vi "videotest.vi"() -> ()   [LabVIEW 2014]
uses:
  <vilib>/userdefined/High Color/IMAQdx.ctl
  <vilib>/vision/driver/NI_Vision_Acquisition_Software.lvlib
panel:
  out "error out":errorcluster
  out "Image":T1(plugin-control)
  in  "stop":bool
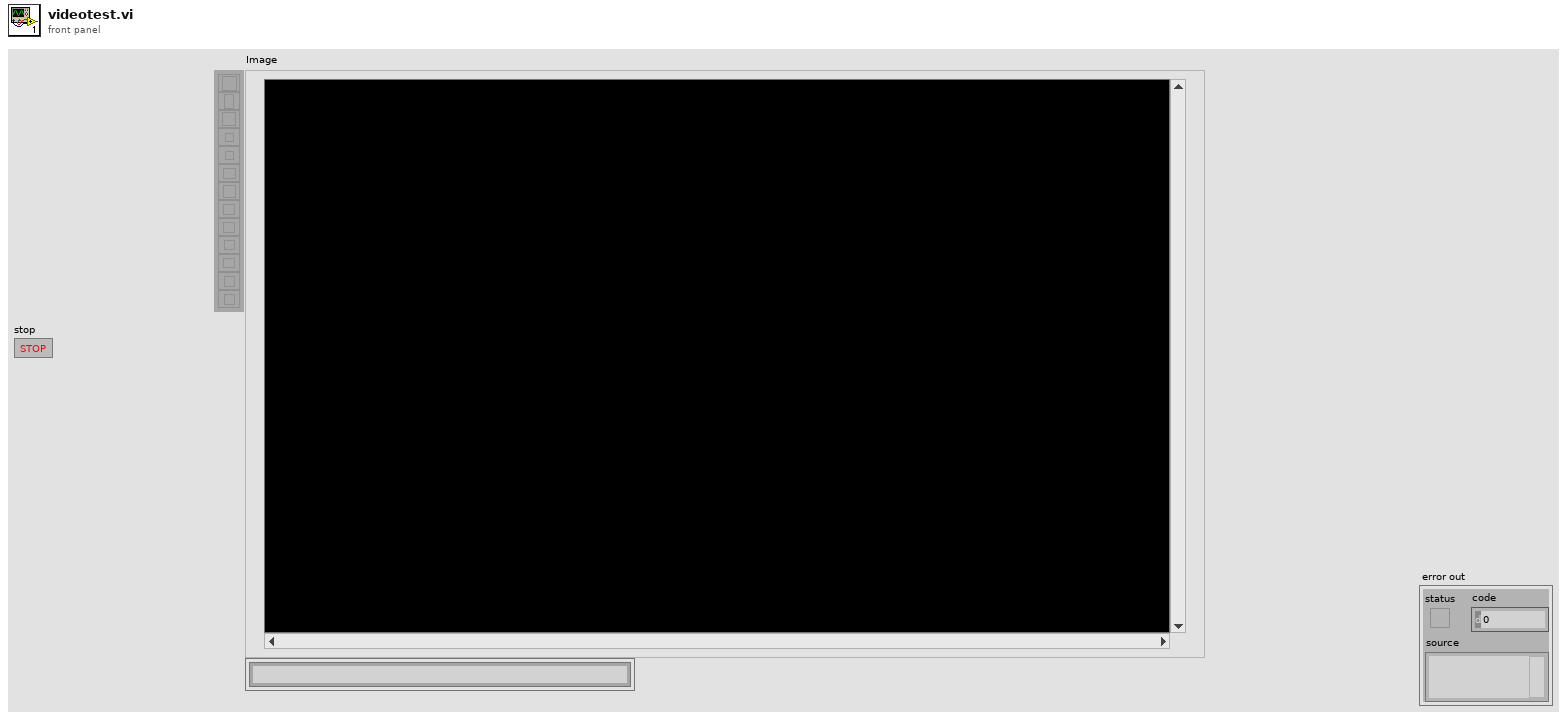
[diagram p1: front panel]
types:
  T1 = typedef "IMAQ Image.ctl" = refnum<image>
  T2 = typedef "IMAQdx.ctl" = refnum<k21>
  T3 = typedef "Image Type" = u32
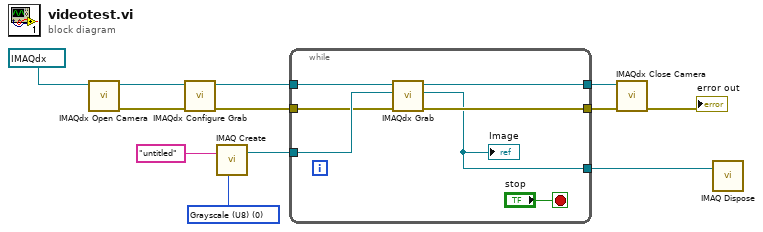
[diagram p0: block diagram]
diagram:
  w5 = T3 0 items=["Grayscale (U8)", "Grayscale (I16)", "Grayscale (SGL)", "Complex (CSG)", "RGB (U32)", "HSL (U32)", "RGB (U64)", "Grayscale (U16)"] ("Image Type")
  n1 = call <vilib>:"IMAQdx Open Camera.vi"("Session In"=T2 "cam0") -> ("error out"=w10:errorcluster, "Session Out"=w8:T2)  [unwired: 9 in]
  n2 = call <vilib>:"IMAQdx Configure Grab.vi"("error in"=w10, "Session In"=w8) -> ("error out"=w9:errorcluster, "Session Out"=w7:T2)  [unwired: 8 in]
  n3 = call "IMAQ Create"("Image Name"="untitled", "Image Type"=w5) -> ("New Image"=w12:T1)  [unwired: 3 in, 1 out]
  n4 = while {
    tunnel: w12 -> [w17]
    tunnel: w7 -> [w18]
    tunnel: w9 -> [w16]
    tunnel: [w15] -> w4
    tunnel: [w14] -> w3
    tunnel: [w13] -> w1
    stop <- "stop" stop-if-true
    n5 = call <vilib>:"IMAQdx Grab.vi"("error in"=w16, "Image In"=w17, "Session In"=w18) -> ("error out"=w15:errorcluster, "Image Out"=w13:T1, "Session Out"=w14:T2)  [unwired: 5 in, 1 out]
    "Image" <- w13
  }
  n6 = call <vilib>:"IMAQdx Close Camera.vi"("error in"=w4, "Session In"=w3) -> ("error out"=→"error out":errorcluster)  [unwired: 9 in]
  n7 = call "IMAQ Dispose"("Image"=w1) -> ()  [unwired: 5 in, 1 out]
